vi "SecondaryData_Example.vi"(9 "Variant":variant, 10 "Input":dbl[](array[numeric]), 11 "Index":i32) -> (2 "SecondaryData":dbl[](array[numeric]))   [LabVIEW 2012]
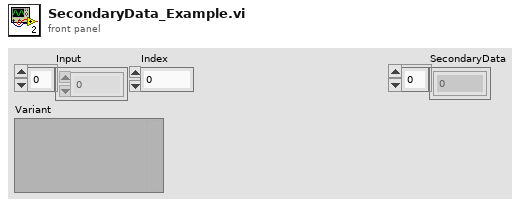
[diagram p1: front panel]
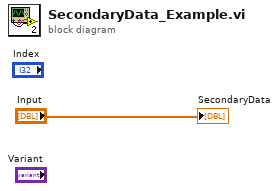
[diagram p0: block diagram]
diagram:
  "SecondaryData" <- "Input"
